vi "DataFinder_Pass_Fail_Analysis.vi"() -> ()   [LabVIEW 2023]
doc: "This example gives you an overview of the DataFinder VIs and shows you how to use the VIs to search in descriptive information on measurement data and to evaluate your search results. For the evaluation, the example displays custom properties of the search results and graphically displays the mass data.\n\nRun the example, execute several queries, receive detailed informations about the search results, and click the stop button to exit."
uses:
  <vilib>/DataFinder/DataTypes/object type.ctl
  <vilib>/DataFinder/DataTypes/comparison operator.ctl
  <vilib>/userdefined/High Color/DFDataFinder.ctl
  <vilib>/DataFinder/Create Query (String).vi
  <vilib>/DataFinder/Create Query (Numeric).vi
  <vilib>/DataFinder/Close Reference (Query).vi
  <vilib>/DataFinder/Create Query (Date).vi
  <vilib>/DataFinder/Close Reference (DataFinder).vi
  <vilib>/DataFinder/NI_DataFinder.lvlib
  <vilib>/userdefined/NI_DataFinder Controls.lvlib
panel:
  in  "DataFinder":T1
  in  "Information":bool
  in  "DisplaySignals":bool
  in  "SearchSensorType":bool
  in  "SearchCalibrationDate":bool
  out "Search Results":string[][](table) caption="Search Results (5)"
  out "Object Type 4":T2=2 items=["File", "Channel Group", "Channel"]
  out "Property Name 4":string="Maximum"
  in  "Value 4":dbl=45.0
  in  "Operator 4":T3=2 items=["=", "<>", ">", "<", ">=", "<=", "#"]
  out "Object Type 3":T2=1 items=["File", "Channel Group", "Channel"]
  out "Property Name 3":string="Test_Status"
  in  "Value 3":string(combo)="Fail"
  out "Operator 3":T3 items=["=", "<>", ">", "<", ">=", "<=", "#"]
  out "Object Type 2":T2=1 items=["File", "Channel Group", "Channel"]
  out "Property Name 2":string="name"
  out "Value 2":string="*Lower*"
  out "Operator 2":T3 items=["=", "<>", ">", "<", ">=", "<=", "#"]
  in  "Stop Button":bool
  out "Object Type":T2 items=["File", "Channel Group", "Channel"]
  out "Property Name":string="fileName"
  out "Value":string="TR_M17_QT_*"
  in  "Search":bool
  out "Operator":T3 items=["=", "<>", ">", "<", ">=", "<=", "#"]
  # "Overview: Executes a predefined query to search for sensor data and analyze the search results.\nRequirements: Select a registered DataFinder which has indexed the TDM Server Demo Data and has optimized the custom properties.\nInstructions:\n1. Ensure that the selected DataFinder is already running.\n2. Run the VI.\n3. Change the Test_Status of the channel group or channel maximum to find failed and passed measurements with certain limits.\n4. In the results table select the search results you are interested in and analyze the results by clicking one of the accordant buttons.\n5. For more information about this example click the Information button.\n6. Click Stop to stop the VI."
  # "Object Type"
  # "Property Name"
  # "Operator"
  # "Value"
  # "Analyze Selected Results"
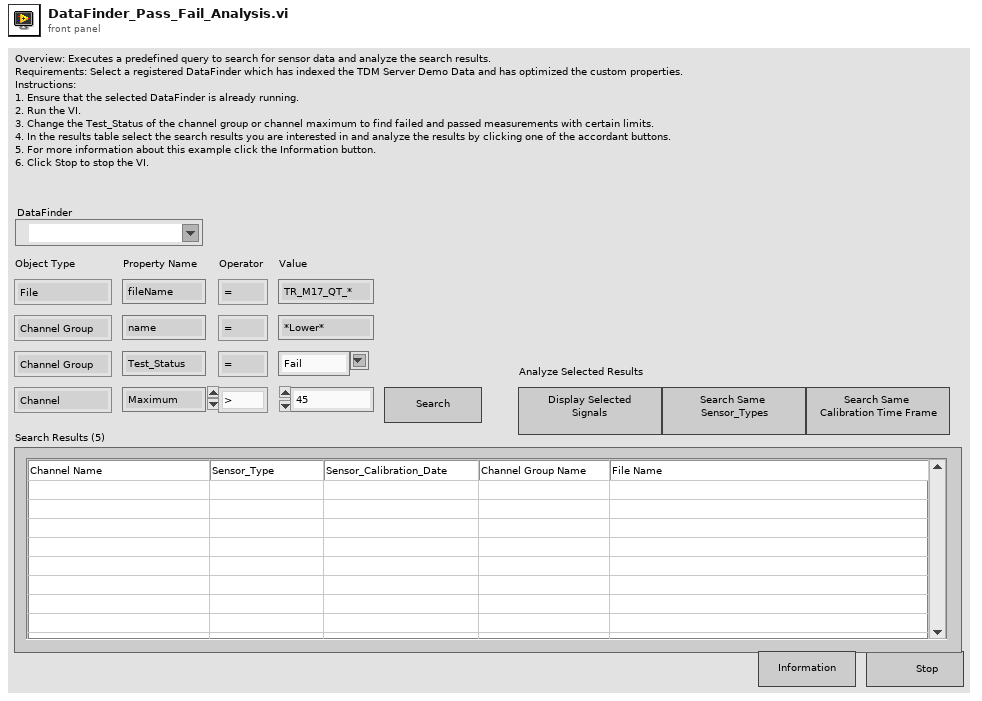
[diagram p1: front panel]
types:
  T1 = typedef "NI_DataFinder Controls.lvlib/DFDataFinder.ctl" = refnum<k21>
  T2 = typedef "NI_DataFinder.lvlib/object type.ctl" = u16
  T3 = typedef "NI_DataFinder.lvlib/comparison operator.ctl" = u16
  T4 = typedef "NI_DataFinder Controls.lvlib/DFQuery.ctl" = refnum<k20>
  T5 = typedef "NI_DataFinder Controls.lvlib/DFSearchResult.ctl" = refnum<k20>
  T6 = typedef "NI_DataFinder.lvlib/results elements.ctl" = cluster{"fullpaths":path[], "DataPlugin names":string[], "channel group names":string[], "channel names":string[]}
  T7 = typedef "LVRowAndColumnTypeDef.ctl" = cluster{"Row":i32, "Column":i32}
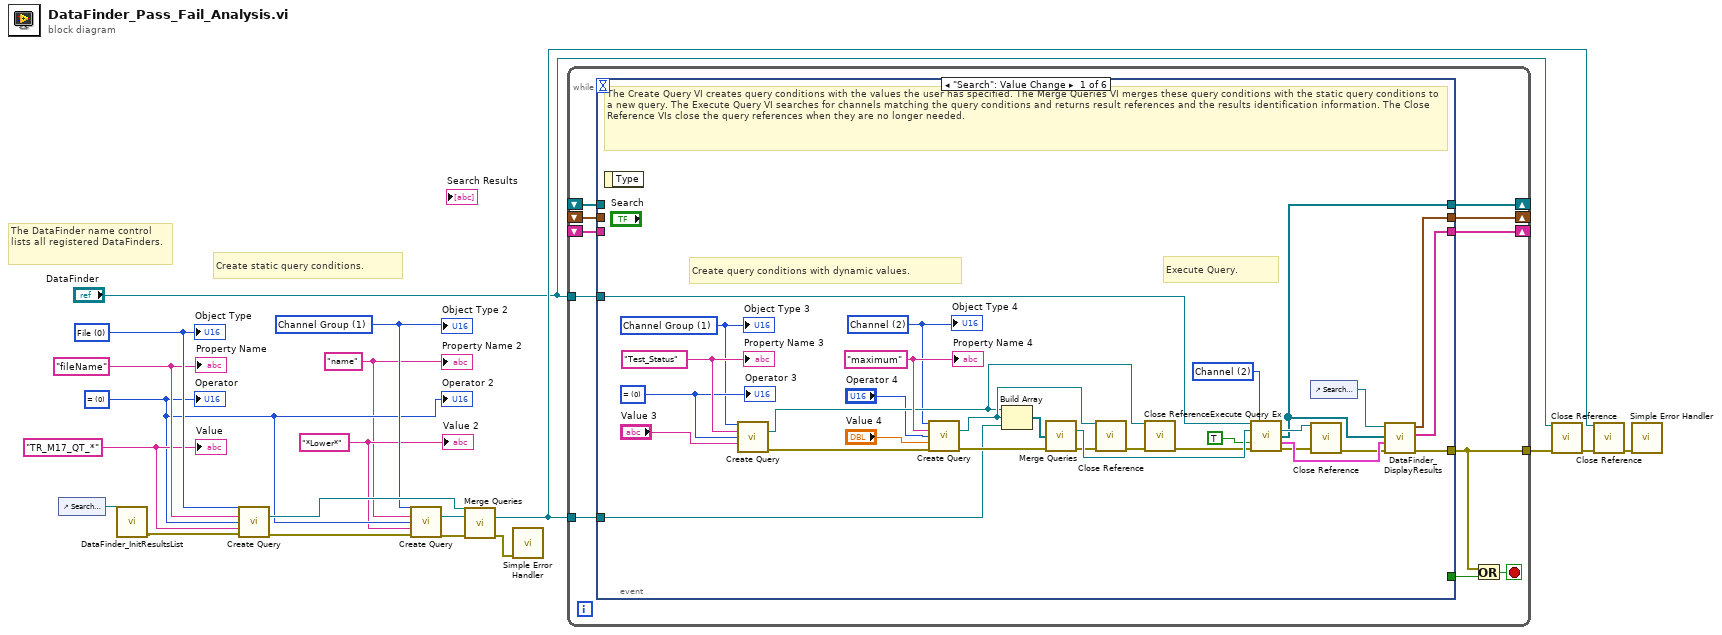
[diagram p0: block diagram]
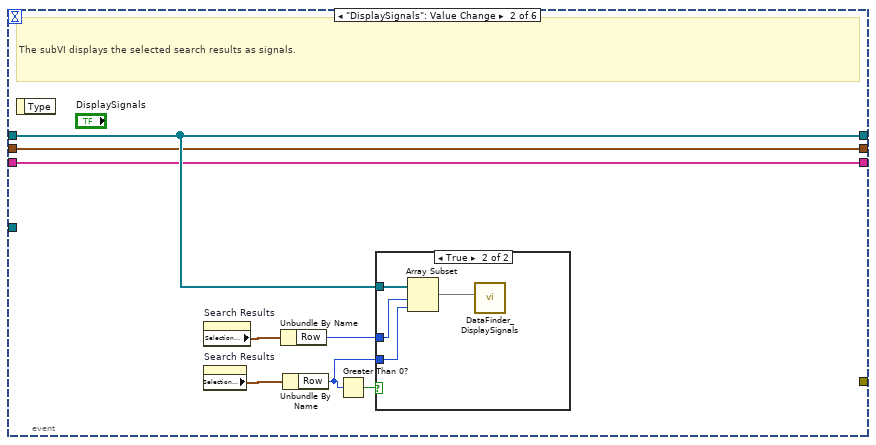
[diagram p2: hidden frame]
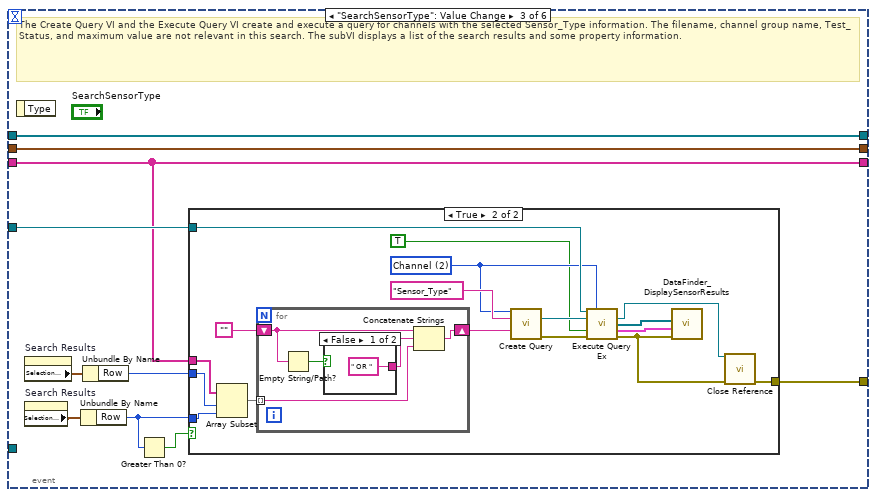
[diagram p4: hidden frame]
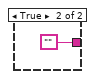
[diagram p6: hidden frame]
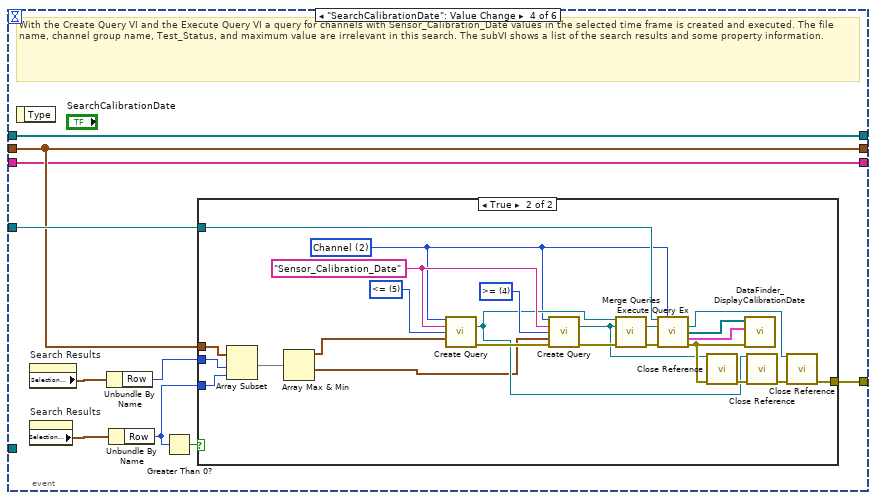
[diagram p7: hidden frame]
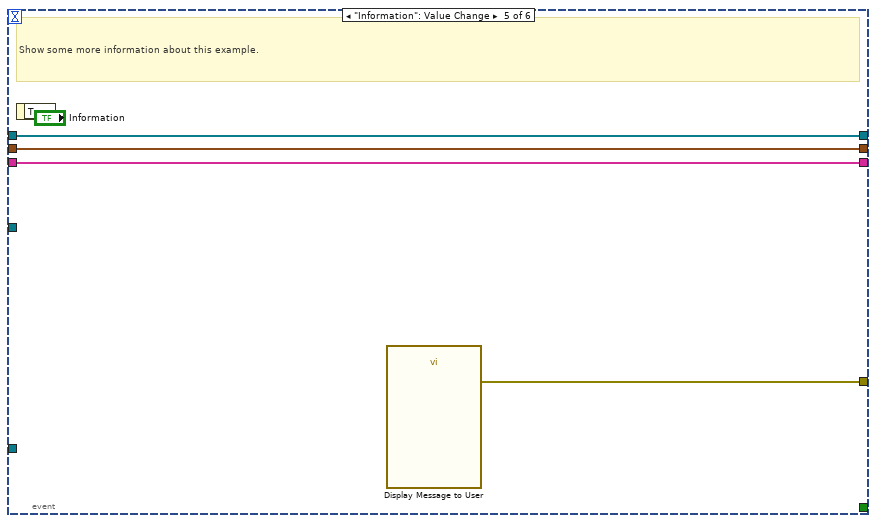
[diagram p9: hidden frame]
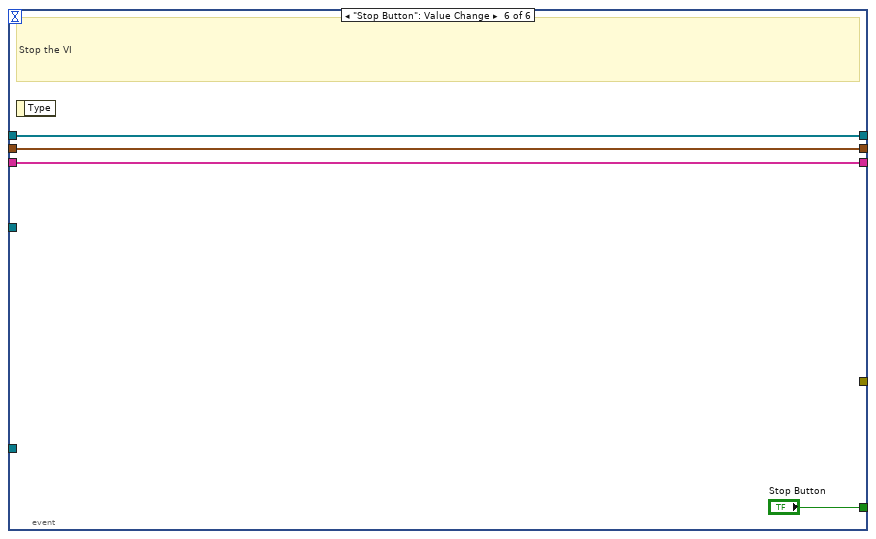
[diagram p10: hidden frame]
diagram:
  w9 = "*Lower*" ("Value 2")
  w8 = "name" ("Property Name 2")
  w11 = T2 1 items=["File", "Channel Group", "Channel"] ("Object Type 2")
  w12 = "TR_M17_QT_*" ("Value")
  w10 = T3 0 items=["=", "<>", ">", "<", ">=", "<=", "#"] ("Operator")
  w13 = "fileName" ("Property Name")
  w14 = T2 0 items=["File", "Channel Group", "Channel"] ("Object Type")
  # "The DataFinder name control lists all registered DataFinders."
  # "Create static query conditions."
  n1 = control-ref of="Search Results"() -> (w15:refnum<vi>)
  n2 = call "DataFinder_InitResultsList.vi"("Tbl Refnum"=w15) -> ("error out"=w1:errorcluster)  [unwired: 10 out]
  n3 = call-poly <vilib>:"Create Query.vi"("object type"=w14, "property name"=w13, "comparison operator (=)"=w10, "value"=w12, "error in (no error)"=w1) -> ("query reference out"=w18:T4, "error out"=w19:errorcluster)  [unwired: 9 in]
  n4 = call-poly <vilib>:"Create Query.vi"("object type"=w11, "property name"=w8, "comparison operator (=)"=w10, "value"=w9, "error in (no error)"=w19) -> ("query reference out"=w17:T4, "error out"=w16:errorcluster)  [unwired: 9 in]
  n5 = call <vilib>:"Merge Queries.vi"("query reference in 1"=w18, "query reference in 2"=w17, "error in (no error)"=w16) -> ("query reference out"=w3:T4, "error out"=w7:errorcluster)  [unwired: 11 in]
  n6 = call <vilib>:"Simple Error Handler.vi"("error in (no error)"=w7) -> ()  [unwired: 4 in, 5 out]
  n7 = while {
    tunnel: "DataFinder" -> [w30]
    tunnel: w3 -> [w23]
    shift-right: [w29] -> _
    shift-left: _ -> [w28]
    shift-right: [w27] -> _
    shift-left: _ -> [w26]
    shift-right: [w25] -> _
    shift-left: _ -> [w24]
    tunnel: [w20] -> w6
    stop <- w22 stop-if-true
    n8 = event shown="[0] \"Search\": Value Change" {
      selector: _ -> [_ _ _ _ _ _]
      dyn-events: _ -> [_ _ _ _ _ _]
      timeout: _ -> [_ _ _ _ _ _]
      tunnel: [_ _ _ _ _ "Stop Button"] -> w21
      tunnel: w30 -> [w59 _ w79 w115 _ _]
      tunnel: w23 -> [w37 _ _ _ _ _]
      tunnel: [w50 _ w76 w110 w144 _] -> w20
      tunnel: [w47 w62 w74 w109 w142 w146] -> w29
      tunnel: w28 -> [_ w62 w74 w109 w142 w146]
      tunnel: [w46 w61 w73 w107 w141 w145] -> w27
      tunnel: w26 -> [_ w61 w73 w107 w141 w145]
      tunnel: [w45 w63 w75 w108 w143 w147] -> w25
      tunnel: w24 -> [_ w63 w75 w108 w143 w147]
      event "Search": Value Change {
        w34 = T2 1 items=["File", "Channel Group", "Channel"] ("Object Type 2")
        w35 = T2 2 items=["File", "Channel Group", "Channel"] ("Object Type 2")
        w36 = T2 2 items=["File", "Channel Group", "Channel"] ("Object Type 2")
        w53 = T3 0 items=["=", "<>", ">", "<", ">=", "<=", "#"] ("Operator 3")
        w52 = "maximum" ("Property Name 4")
        w54 = "Test_Status" ("Property Name 3")
        # "Execute Query."
        # "Create query conditions with dynamic values."
        # "The Create Query VI creates query conditions with the values the user has specified. The Merge Queries VI merges these query conditions with the static query conditions to a new query. The Execute Query VI searches for channels matching the query conditions and returns result references and the results identification information. The Close Reference VIs close the query references when they are no longer needed."
        n9 = event-data() -> ()  [unwired: 2 out]
        n10 = call-poly <vilib>:"Create Query.vi"("object type"=w34, "property name"=w54, "comparison operator (=)"=w53, "value"="Value 3") -> ("query reference out"=w38:T4, "error out"=w58:errorcluster)  [unwired: 10 in]
        n11 = call-poly <vilib>:"Create Query.vi"("object type"=w35, "property name"=w52, "comparison operator (=)"="Operator 4", "value"="Value 4", "error in (no error)"=w58) -> ("query reference out"=w39:T4, "error out"=w56:errorcluster)  [unwired: 9 in]
        n12 = Build Array(w38, w39, w37) -> (w44:T4[])
        n13 = call <vilib>:"Merge Queries.vi"("query reference array in"=w44, "error in (no error)"=w56) -> ("query reference out"=w55:T4, "error out"=w42:errorcluster)  [unwired: 12 in]
        n14 = call-poly <vilib>:"Close Reference.vi"("query reference"=w39, "error in (no error)"=w42) -> ("error out"=w41:errorcluster)  [unwired: 13 in]
        n15 = call-poly <vilib>:"Close Reference.vi"("query reference"=w38, "error in (no error)"=w41) -> ("error out"=w40:errorcluster)  [unwired: 13 in]
        n16 = call <vilib>:"Execute Query Ex.vi"("DataFinder reference"=w59, "result object type (file)"=w36, "query reference"=w55, "fill results elements? (F)"=TRUE, "error in (no error)"=w40) -> ("query reference out"=w49:T4, "result references out"=w45:T5[], "results elements"=w60:T6, "error out"=w48:errorcluster)  [unwired: 5 in, 2 out]
        n17 = control-ref of="Search Results"() -> (w51:refnum<vi>)
        n18 = call-poly <vilib>:"Close Reference.vi"("query reference"=w49, "error in (no error)"=w48) -> ("error out"=w43:errorcluster)  [unwired: 13 in]
        n19 = call "DataFinder_DisplayResults.vi"("error in"=w43, "results elements"=w60, "result references"=w45, "Tbl Refnum"=w51) -> ("error out"=w50:errorcluster, "Sensor_Type values"=w46:string[], "Calibration_Date values"=w47:timestamp[])  [unwired: 5 in]
        "Property Name 3" <- w54
        "Property Name 4" <- w52
        "Object Type 4" <- w35
        "Object Type 3" <- w34
        "Operator 3" <- w53
      }
      event "DisplaySignals": Value Change {
        # "The subVI displays the selected search results as signals."
        n20 = event-data() -> ()  [unwired: 2 out]
        n21 = property on="Search Results" class="Tbl (strict)"() -> ("Selection Start"=w68:T7)  [unwired: 2 in, 2 out]
        n22 = property on="Search Results" class="Tbl (strict)"() -> ("Selection Size"=w67:T7)  [unwired: 2 in, 2 out]
        n23 = Unbundle By Name(w68) -> ("Row"=w65:i32)
        n24 = Unbundle By Name(w67) -> ("Row"=w64:i32)
        n25 = Greater Than 0?(x=w64) -> (x > 0?=w66:bool)
        n26 = case shown="True" w66 {
          tunnel: w63 -> [_ w72]
          tunnel: w65 -> [_ w71]
          tunnel: w64 -> [_ w70]
          frame False {
          }
          frame True {
            n27 = Array Subset(array=w72, index=w71, length=w70) -> (w69:T5[])
            n28 = call "DataFinder_DisplaySignals.vi"("result references"=w69) -> ()  [unwired: 11 in]
          }
        }
      }
      event "SearchSensorType": Value Change {
        # "The Create Query VI and the Execute Query VI create and execute a query for channels with the selected Sensor_Type information. The filename, channel group name, Test_Status, and maximum value are not relevant in this search. The subVI displays a list of the search results and some property information."
        n29 = event-data() -> ()  [unwired: 2 out]
        n30 = property on="Search Results" class="Tbl (strict)"() -> ("Selection Start"=w82:T7)  [unwired: 2 in, 2 out]
        n31 = property on="Search Results" class="Tbl (strict)"() -> ("Selection Size"=w80:T7)  [unwired: 2 in, 2 out]
        n32 = Unbundle By Name(w80) -> ("Row"=w78:i32)
        n33 = Unbundle By Name(w82) -> ("Row"=w81:i32)
        n34 = Greater Than 0?(x=w78) -> (x > 0?=w77:bool)
        n35 = case shown="True" w77 {
          tunnel: w81 -> [_ w99]
          tunnel: w73 -> [_ w98]
          tunnel: w79 -> [_ w91]
          tunnel: w78 -> [_ w89]
          tunnel: [_ w87] -> w76
          frame False {
          }
          frame True {
            w84 = T2 2 items=["File", "Channel Group", "Channel"] ("Object Type 2")
            n36 = Array Subset(array=w98, index=w99, length=w89) -> (w97:string[])
            n37 = for {
              tunnel: w97 -> [w100] mode=indexing
              shift-right: [w101] -> w94
              shift-left: "" -> [w104]
              n38 = Empty String/Path?(string/path=w104) -> (empty?=w103:bool)
              n39 = case shown="False" w103 {
                tunnel: [" OR " ""] -> w102
                frame False {
                }
                frame True {
                }
              }
              n40 = Concatenate Strings(w104, w102, w100) -> (w101:string)
            }
            n41 = call-poly <vilib>:"Create Query.vi"("object type"=w84, "property name"="Sensor_Type", "value"=w94) -> ("query reference out"=w93:T4, "error out"=w92:errorcluster)  [unwired: 11 in]
            n42 = call <vilib>:"Execute Query Ex.vi"("DataFinder reference"=w91, "result object type (file)"=w84, "query reference"=w93, "fill results elements? (F)"=TRUE, "error in (no error)"=w92) -> ("query reference out"=w85:T4, "result references out"=w90:T5[], "results elements"=w88:T6, "error out"=w86:errorcluster)  [unwired: 5 in, 2 out]
            n43 = call "DataFinder_DisplaySensorResults.vi"("result references"=w90, "results elements"=w88, "error in"=w86) -> ()  [unwired: 8 in]
            n44 = call-poly <vilib>:"Close Reference.vi"("query reference"=w85, "error in (no error)"=w86) -> ("error out"=w87:errorcluster)  [unwired: 13 in]
          }
        }
      }
      event "SearchCalibrationDate": Value Change {
        # "With the Create Query VI and the Execute Query VI a query for channels with Sensor_Calibration_Date values in the selected time frame is created and executed. The file name, channel group name, Test_Status, and maximum value are irrelevant in this search. The subVI shows a list of the search results and some property information."
        n45 = event-data() -> ()  [unwired: 2 out]
        n46 = property on="Search Results" class="Tbl (strict)"() -> ("Selection Start"=w114:T7)  [unwired: 2 in, 2 out]
        n47 = property on="Search Results" class="Tbl (strict)"() -> ("Selection Size"=w113:T7)  [unwired: 2 in, 2 out]
        n48 = Unbundle By Name(w114) -> ("Row"=w116:i32)
        n49 = Unbundle By Name(w113) -> ("Row"=w111:i32)
        n50 = Greater Than 0?(x=w111) -> (x > 0?=w112:bool)
        n51 = case shown="True" w112 {
          tunnel: w109 -> [_ w132]
          tunnel: w116 -> [_ w133]
          tunnel: w115 -> [_ w135]
          tunnel: w111 -> [_ w134]
          tunnel: [_ w125] -> w110
          frame False {
          }
          frame True {
            w117 = T2 2 items=["File", "Channel Group", "Channel"] ("object type")
            w138 = T3 4 items=["=", "<>", ">", "<", ">=", "<=", "#"] ("comparison operator (=)")
            w140 = T3 5 items=["=", "<>", ">", "<", ">=", "<=", "#"] ("comparison operator (=)")
            w139 = "Sensor_Calibration_Date" ("property name")
            n52 = Array Subset(array=w132, index=w133, length=w134) -> (w120:timestamp[])
            n53 = Array Max & Min(array=w120) -> (max value=w119:timestamp, min value=w118:timestamp)  [unwired: 2 out]
            n54 = call-poly <vilib>:"Create Query.vi"("object type"=w117, "property name"=w139, "comparison operator (=)"=w140, "value"=w119) -> ("query reference out"=w121:T4, "error out"=w131:errorcluster)  [unwired: 10 in]
            n55 = call-poly <vilib>:"Create Query.vi"("object type"=w117, "property name"=w139, "comparison operator (=)"=w138, "value"=w118, "error in (no error)"=w131) -> ("query reference out"=w122:T4, "error out"=w130:errorcluster)  [unwired: 9 in]
            n56 = call <vilib>:"Merge Queries.vi"("query reference in 1"=w121, "query reference in 2"=w122, "error in (no error)"=w130) -> ("query reference out"=w137:T4, "error out"=w136:errorcluster)  [unwired: 11 in]
            n57 = call <vilib>:"Execute Query Ex.vi"("DataFinder reference"=w135, "result object type (file)"=w117, "query reference"=w137, "error in (no error)"=w136) -> ("query reference out"=w123:T4, "result references out"=w128:T5[], "results elements"=w129:T6, "error out"=w124:errorcluster)  [unwired: 6 in, 2 out]
            n58 = call-poly <vilib>:"Close Reference.vi"("query reference"=w122, "error in (no error)"=w124) -> ("error out"=w127:errorcluster)  [unwired: 13 in]
            n59 = call "DataFinder_DisplayCalibrationDate.vi"("error in"=w124, "results elements"=w129, "result references"=w128) -> ()  [unwired: 9 in]
            n60 = call-poly <vilib>:"Close Reference.vi"("query reference"=w121, "error in (no error)"=w127) -> ("error out"=w126:errorcluster)  [unwired: 13 in]
            n61 = call-poly <vilib>:"Close Reference.vi"("query reference"=w123, "error in (no error)"=w126) -> ("error out"=w125:errorcluster)  [unwired: 13 in]
          }
        }
      }
      event "Information": Value Change {
        # "Show some more information about this example."
        n62 = event-data() -> ()  [unwired: 2 out]
        n63 = call "Display Message to User"() -> ("error out"=w144:errorcluster)  [unwired: 10 in, 1 out]
      }
      event "Stop Button": Value Change {
        # "Stop the VI"
        n64 = event-data() -> ()  [unwired: 2 out]
      }
    }
    n65 = Or(x=w20, y=w21) -> (x .or. y?=w22:bool)
  }
  n66 = call-poly <vilib>:"Close Reference.vi"("DataFinder reference"="DataFinder", "error in (no error)"=w6) -> ("error out"=w4:errorcluster)  [unwired: 13 in]
  n67 = call-poly <vilib>:"Close Reference.vi"("query reference"=w3, "error in (no error)"=w4) -> ("error out"=w5:errorcluster)  [unwired: 13 in]
  n68 = call <vilib>:"Simple Error Handler.vi"("error in (no error)"=w5) -> ()  [unwired: 4 in, 5 out]
  "Object Type" <- w14
  "Property Name" <- w13
  "Operator" <- w10
  "Operator 2" <- w10
  "Value 2" <- w9
  "Property Name 2" <- w8
  "Object Type 2" <- w11
  "Value" <- w12
